vi "UpdateMethodSignatureText.vi"(10 "TagCodedStringIn":string) -> (2 "StringOut":string)   [LabVIEW 2020, in "ClassWriterNative.lvclass"]
uses:
  <resource>/Framework/Providers/Open_GDS/ClassProviders/Provider_LvNativeClass/ClassWriterNative_class/ClassWriterNative.lvclass
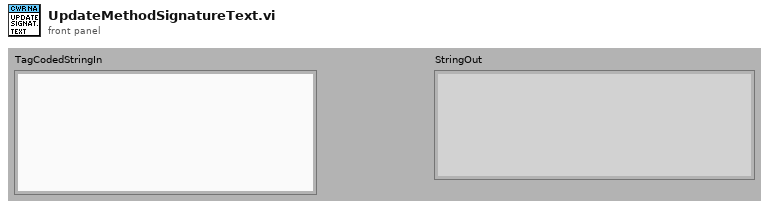
[diagram p1: front panel]
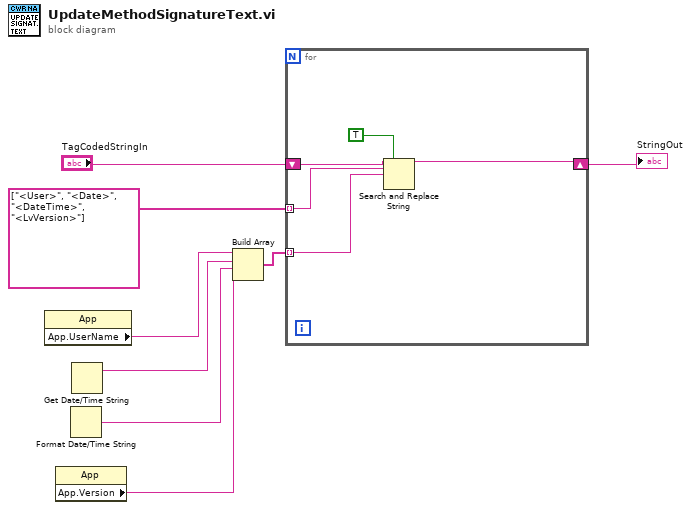
[diagram p0: block diagram]
diagram:
  n1 = property class="App"() -> ("App.UserName"=w4:string)  [unwired: 2 in, 2 out]
  n2 = property class="App"() -> ("App.Version"=w1:string)  [unwired: 2 in, 2 out]
  n3 = Format Date/Time String() -> (date/time string=w2:string)  [unwired: 3 in]
  n4 = Get Date/Time String() -> (date string=w3:string)  [unwired: 3 in, 1 out]
  n5 = Build Array(w4, w3, w2, w1) -> (w5:string[])
  n6 = for {
    shift-right: [w11] -> w7
    shift-left: "TagCodedStringIn" -> [w13]
    tunnel: string[] ["<User>", "<Date>", "<DateTime>", "<LvVersion>"] -> [w10] mode=indexing
    tunnel: w5 -> [w9] mode=indexing
    n7 = Search and Replace String(replace all?=TRUE ("replace all? (F)"), input string=w13, search string=w10, replace string=w9) -> (result string=w11:string)  [unwired: 4 in, 3 out]
  }
  "StringOut" <- w7
